vi "encodeUInt8.vi"(2 "Compress? (T)":bool=TRUE, 3 "UInt8":u8) -> (1 "MessagePack":u8[](array[numeric]) format="%.0x")   [LabVIEW 2015, in "MsgPack.lvlib"]
uses:
  MsgPack.lvlib
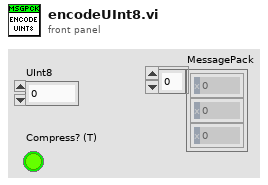
[diagram p1: front panel]
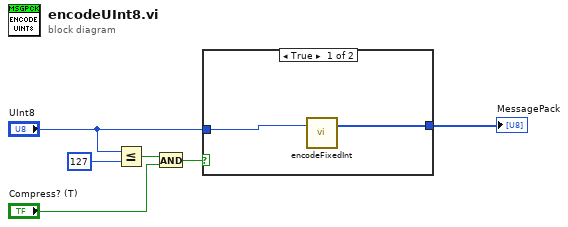
[diagram p0: block diagram]
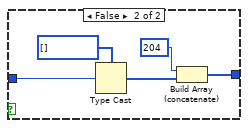
[diagram p2: hidden frame]
diagram:
  n1 = Less Or Equal?(x="UInt8", y=u8 127) -> (x <= y?=w4:bool)
  n2 = And(x=w4, y="Compress? (T)") -> (x .and. y?=w2:bool)
  n3 = case shown="True" w2 {
    tunnel: [w7 w13] -> w6
    tunnel: "UInt8" -> [w8 w9]
    frame True {
      n4 = call "encodeFixedInt.vi"("FixedInt8"=w8) -> ("Array"=w7:u8[])  [unwired: 2 in]
    }
    frame False {
      n5 = Type Cast(type=u8[] [], x=w9) -> (*(type *) &x=w10:u8[])
      n6 = Build Array (concatenate)(u8 204, w10) -> (w13:u8[])
    }
  }
  "MessagePack" <- w6
